vi "DeCoF get trace from binary.vi"(2 "Block ID":string="Y", 3 "Binary in":string) -> (0 "float array":sgl[](array[numeric]))   [LabVIEW 2013]
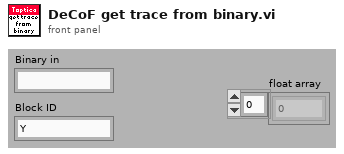
[diagram p1: front panel]
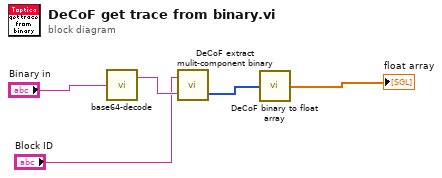
[diagram p0: block diagram]
diagram:
  n1 = call "base64-decode.vi"("String"="Binary in") -> ("binary output"=w5:string)  [unwired: 1 out]
  n2 = call "DeCoF extract mulit-component binary.vi"("decoded binary blob"=w5, "identifier"="Block ID") -> ("bytes"=w4:u8[])  [unwired: 1 out]
  n3 = call "DeCoF binary to float array.vi"("byte buffer"=w4) -> ("float array"=→"float array":sgl[])
